vi "CtrProps.vi"(10 "error in (no error)":errorcluster, 11 ".NET Refnum 2":refnum<k24>) -> (0 "InitialState":i32, 1 "ClearOnRead":bool, 2 "error out":errorcluster, 3 ".NET Refnum":refnum<k24>)   [LabVIEW 2010]
uses:
  C:/Program Files/National Instruments/LabVIEW 2010/vi.lib/ULx/ULx_LV.dll
  Program Files/National Instruments/LabVIEW 2010/vi.lib/ULx/ULx_LV.dll
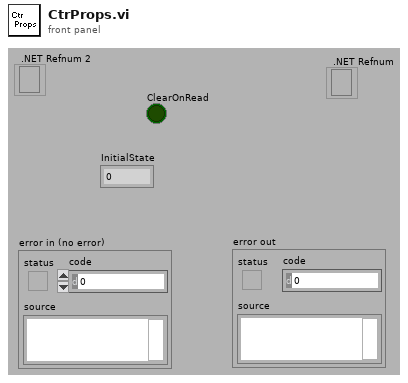
[diagram p1: front panel]
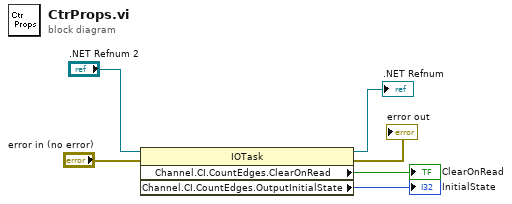
[diagram p0: block diagram]
diagram:
  n1 = property class="IOTask"(reference=".NET Refnum 2", error in="error in (no error)") -> (reference out=→".NET Refnum":refnum<k24>, error out=→"error out":errorcluster, "Channel.CI.CountEdges.ClearOnRead"=→"ClearOnRead":bool, "Channel.CI.CountEdges.OutputInitialState"=→"InitialState":i32)
